vi "Enable LAN Connect State.vi"(8 "error in (no error)":errorcluster, 9 "Enable Connect (F: False)":bool, 10 "LAN Event Number   (1)":i32=1 format="%#.6g", 11 "VISA resource name":refnum<visa-resource-name>) -> (0 "error out":errorcluster, 3 "VISA resource name out":refnum<visa-resource-name>)   [LabVIEW 2021, in "Keithley 2450.lvlib"]
doc: "Enables or Disables out going LAN triggers on an event."
uses:
  <instrlib>/Keithley 2450/Keithley 2450.lvlib
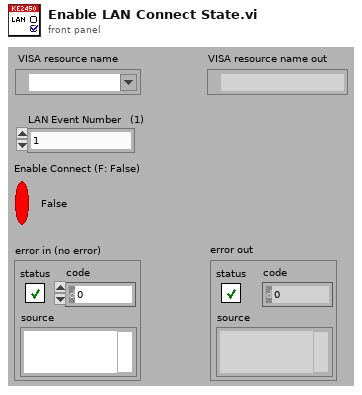
[diagram p1: front panel]
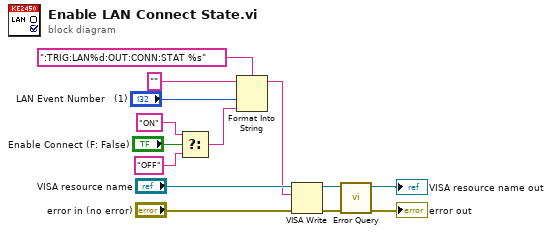
[diagram p0: block diagram]
diagram:
  n1 = Select(t="ON" ("format string"), s="Enable Connect (F: False)", f="OFF" ("format string")) -> (s? t:f=w2:string)
  n2 = Format Into String(format string=":TRIG:LAN%d:OUT:CONN:STAT %s", initial string="", "LAN Event Number   (1)", w2) -> (resulting string=w1:string)  [unwired: 1 in, 1 out]
  n3 = VISA Write(VISA resource name="VISA resource name", write buffer=w1, error in (no error)="error in (no error)") -> (VISA resource name out=w12:refnum<visa-resource-name>, error out=w9:errorcluster)  [unwired: 1 out]
  n4 = call <instrlib>:"Error Query.vi"("error in (no error)"=w9, "VISA resource name"=w12) -> ("error out"=→"error out":errorcluster, "VISA resource name out"=→"VISA resource name out":refnum<visa-resource-name>)  [unwired: 8 out]
